vi "INTRO WINDOW.vi"(9 "Monitor(1)":u16=1, 11 "Loading...":refnum<vi>) -> ()   [LabVIEW 2019]
panel:
  out "INTRO INTESYS":cluster{"Loading...":u8} {"Loading..." scale=0.0..100.0}
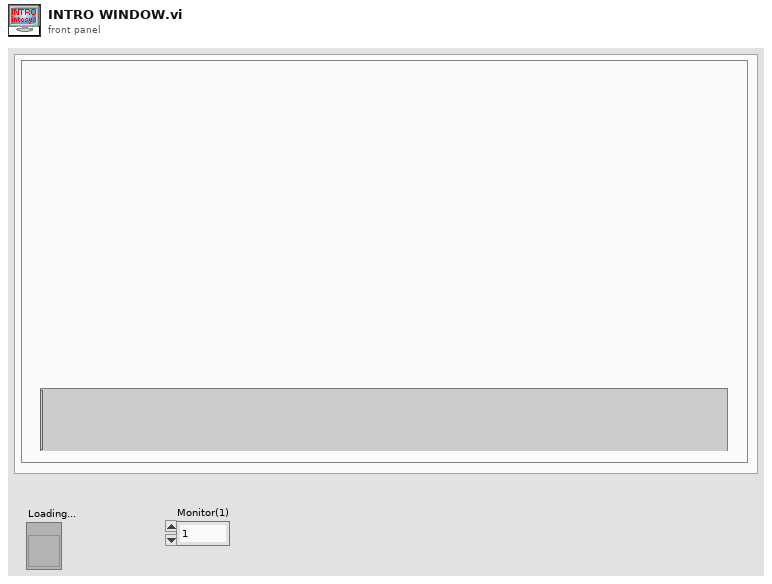
[diagram p1: front panel]
types:
  T1 = enum16{"ALIGN -CENTER", "ALIGN -TOP LEFT", "ALIGN -AS IS", "ALIGN -CUSTOM"}
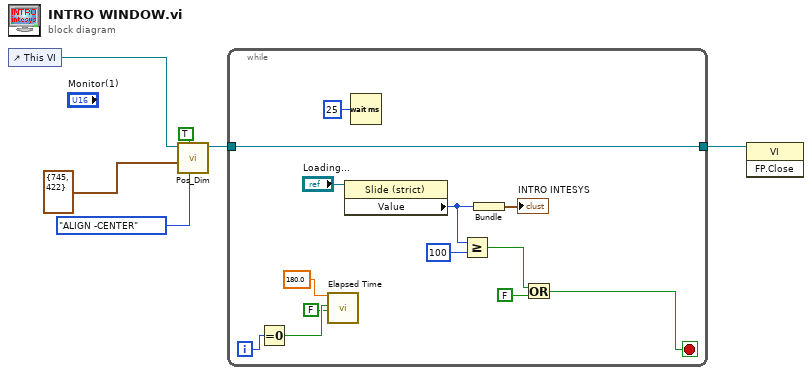
[diagram p0: block diagram]
diagram:
  n1 = control-ref of="This VI"() -> (w6:refnum<vi>)
  n2 = call "Pos_Dim.vi"("Mode"=T1."ALIGN -CENTER", "Open FP"=TRUE, "Size"=cluster{"right":i16, "bottom":i16} {"right"=745, "bottom"=422}, "VIRefNum  IN"=w6) -> ("VIRefNum OUT"=w3:refnum<vi>)  [unwired: 6 in, 1 out]
  n3 = while {
    tunnel: w3 -> [w14]
    tunnel: [w14] -> w2
    i -> [w12]
    stop <- w8 stop-if-true
    n4 = Equal To 0?(x=w12) -> (x = 0?=w11:bool)
    n5 = call "Elapsed Time"("Time Target (s)"=180.0, "Reset"=w11, "Auto Reset"=FALSE) -> ()  [unwired: 9 in, 8 out]
    n6 = property class="Slide (strict)"(reference="Loading...") -> ("Value"=w16:u8)  [unwired: 1 in, 2 out]
    n7 = Wait (ms)(milliseconds to wait=u32 25) -> ()  [unwired: 1 out]
    n8 = Greater Or Equal?(x=w16, y=u8 100) -> (x >= y?=w13:bool)
    n9 = Bundle("Value"=w16) -> (→"INTRO INTESYS":cluster{"Value":u8})  [unwired: 1 in]
    n10 = Or(x=w13, y=FALSE) -> (x .or. y?=w8:bool)
  }
  n11 = invoke class="VI" method="FP.Close"(reference=w2) -> ()  [unwired: 2 in, 3 out]
